vi "setStyle.vi"(8 "Error In":errorcluster, 10 "style":T1 items=["NoBrush"=0, "SolidPattern"=1, "Dense1Pattern"=2, "Dense2Pattern"=3, "Dense3Pattern"=4, "Dense4Pattern"=5, "Dense5Pattern"=6, "Dense6Pattern"=7, "Dense7Pattern"=8, "HorPattern"=9, "VerPattern"=10, "CrossPattern"=11, "BDiagPattern"=12, "FDiagPattern"=13, "DiagCrossPattern"=14, "LinearGradientPattern"=15, "RadialGradientPattern"=16, "ConicalGradientPattern"=17, "TexturePattern"=24], 11 "QBrush In":refnum<class "QBrush.lvclass">) -> (0 "Error Out":errorcluster, 3 "QBrush Out":refnum<class "QBrush.lvclass">)   [LabVIEW 2014, in "QBrush.lvclass"]
doc: "LabVIEW-specific documentation is not yet available. See <b>https://doc.qt.io/qt-5/qbrush.html#setStyle</b>"
uses:
  QBrush.lvclass
  LQ Core/Qt/BrushStyle.ctl
  LQ Core/LQSerialData/LQSerialData.lvclass/LQSerialData.ctl
  LQ Core/LQ Core.lvlib
  LQ Core/LQSerialData/LQSerialData.lvclass
  LQ Core/Qt/Qt.lvlib
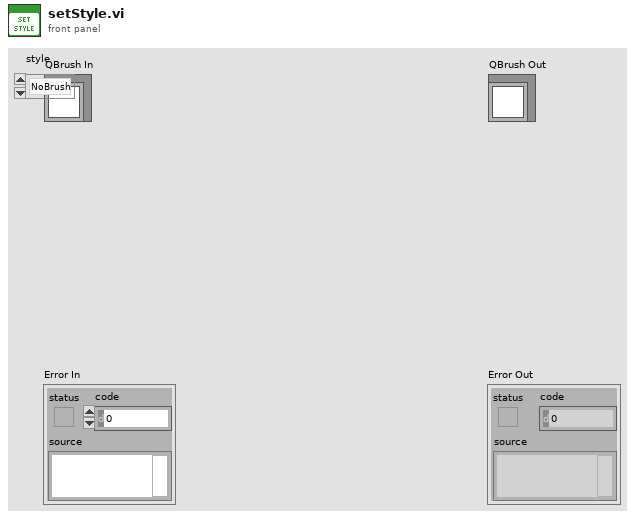
[diagram p1: front panel]
types:
  T1 = typedef "Qt.lvlib/BrushStyle.ctl" = i32
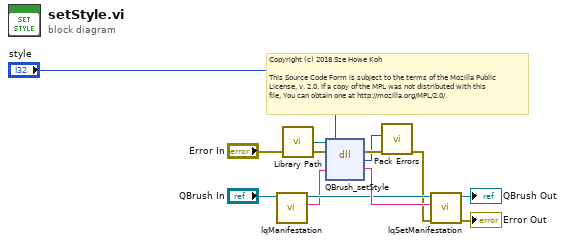
[diagram p0: block diagram]
diagram:
  # "Copyright (c) 2018 Sze Howe Koh\n\nThis Source Code Form is subject to the terms of the Mozilla Public\nLicense, v. 2.0. If a copy of the MPL was not distributed with this\nfile, You can obtain one at http://mozilla.org/MPL/2.0/."
  n1 = call "lqManifestation.vi"("LQSerialData in"="QBrush In") -> ("Manifestation"=w7:string, "LQSerialData out"=w8:refnum<class "QBrush.lvclass">)  [unwired: 9 in]
  n2 = call "Library Path.vi"() -> ("Library Path"=w6:path)
  n3 = dll-call lib="?" fn="QBrush_setStyle"(path in=w6, error in="Error In", "_instance"=w7, "style"="style") -> (error out=w5:errorcluster, w4:i32, "_instance"=w10:string)  [unwired: 2 in, 1 out]
  n4 = call "Pack Errors.vi"("Error In"=w5, "Error Code"=w4) -> ("Error Out"=w3:errorcluster)  [unwired: 9 in]
  n5 = call "lqSetManifestation.vi"("Error In"=w3, "Manifestation"=w10, "LQSerialData in"=w8) -> ("Error Out"=→"Error Out":errorcluster, "LQSerialData out"=→"QBrush Out":refnum<class "QBrush.lvclass">)  [unwired: 7 in]
